vi "XNET.Settings.vi"(6 "Action":enum8{"Get", "Set"}(ring), 8 "error in (no error)":errorcluster, 10 "J1939 XNET Settings":T1={"Database"="", "Cluster"="", "Port"="", "Baud rate [Bd]"=500000, "Termination"=1, "Incoming Decimation"=1, "Outgoing Decimation"=1} {"Termination" items=["Off", "On"]}, 11 "Parent Ref in":T2 format="%.0x") -> (0 "error out":errorcluster, 2 "J1939 XNET Settings":T1={"Database"="", "Cluster"="", "Port"="", "Baud rate [Bd]"=0, "Termination"=0, "Incoming Decimation"=100, "Outgoing Decimation"=100} {"Termination" items=["Off", "On"]}, 3 "Item Ref out":T2 format="%.0x")   [LabVIEW 2019, in "J1939 Addon Shared.lvlib"]
uses:
  J1939 Addon Shared.lvlib
  Constants.vi
  <vilib>/NI VeriStand/Custom Device API/Custom Device API.lvlib
  <vilib>/NI VeriStand/Custom Device API/Get Item Property (String).vi
  <vilib>/NI VeriStand/Custom Device API/Get Item Property (U32).vi
  <vilib>/NI/NI VeriStand Advanced SysDef API/SysDef API/Advanced System Definition.lvlib
  <vilib>/NI/NI VeriStand Advanced SysDef API/_SubVIs/SysDef.Property.Set.String.vi
  <vilib>/NI/NI VeriStand Advanced SysDef API/_SubVIs/SysDef.Property.Set.U32.vi
  Types/XNET Settings.ctl
  <vilib>/NI VeriStand/Custom Device API/Custom Device Item Ref.ctl
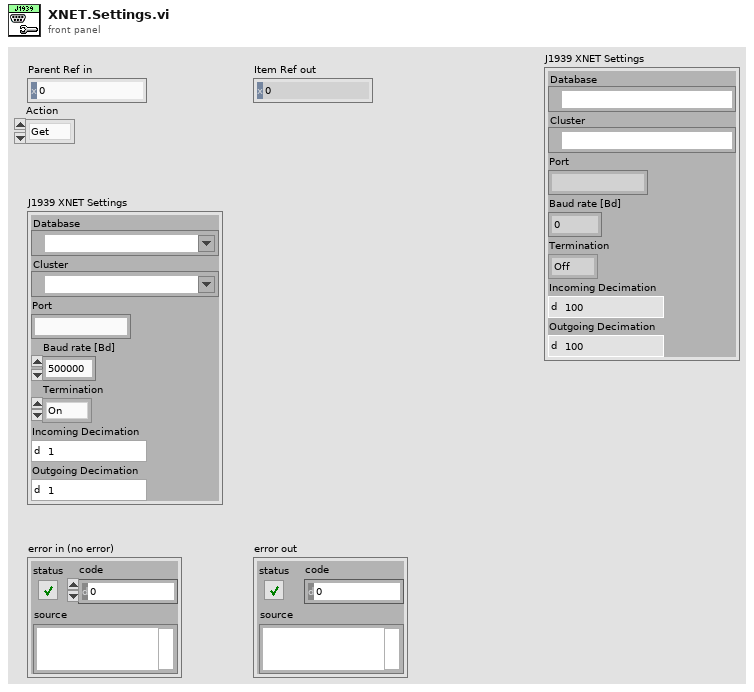
[diagram p1: front panel]
types:
  T1 = typedef "J1939 Addon Shared.lvlib/XNET Settings.ctl" = cluster{"Database":refnum<k21>, "Cluster":refnum<k21>, "Port":string, "Baud rate [Bd]":u32, "Termination":u32, "Incoming Decimation":u32, "Outgoing Decimation":u32}
  T2 = typedef "Custom Device API.lvlib/Custom Device Item Ref.ctl" = u64
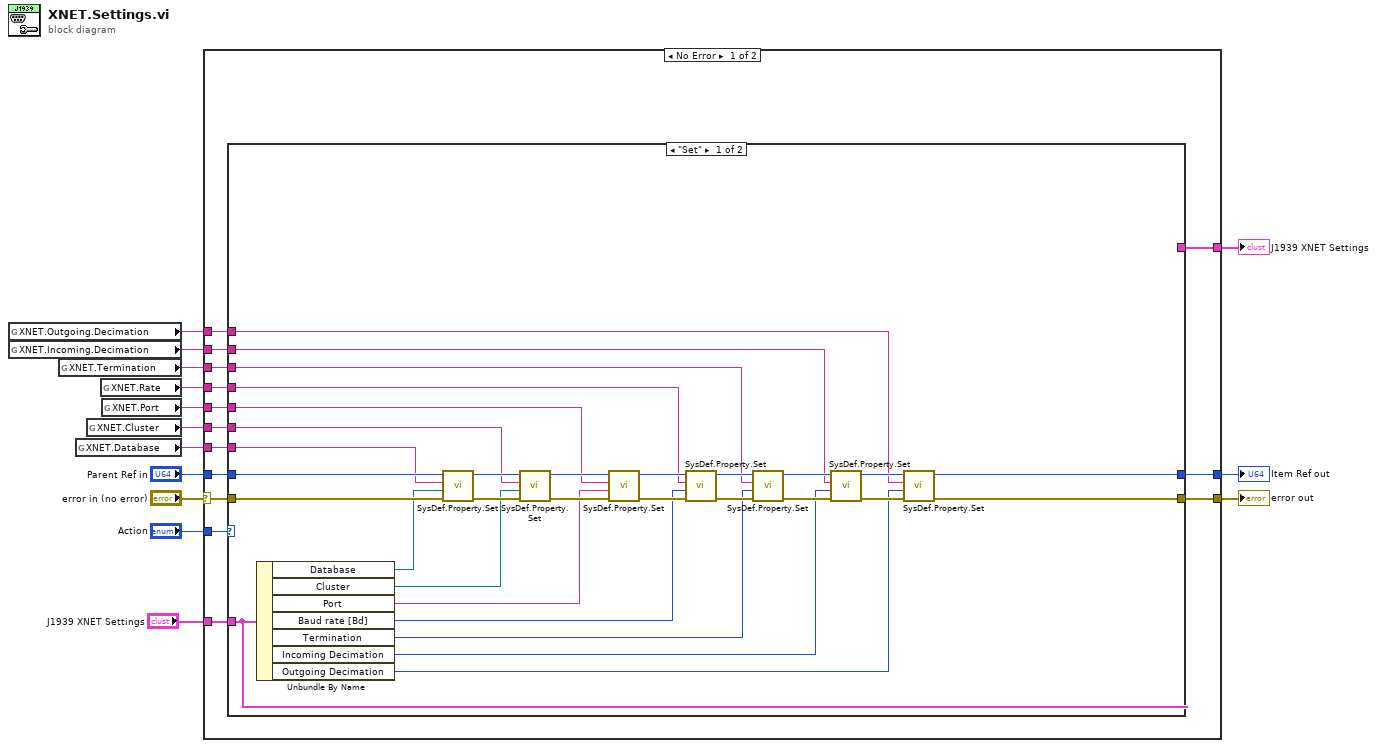
[diagram p0: block diagram]
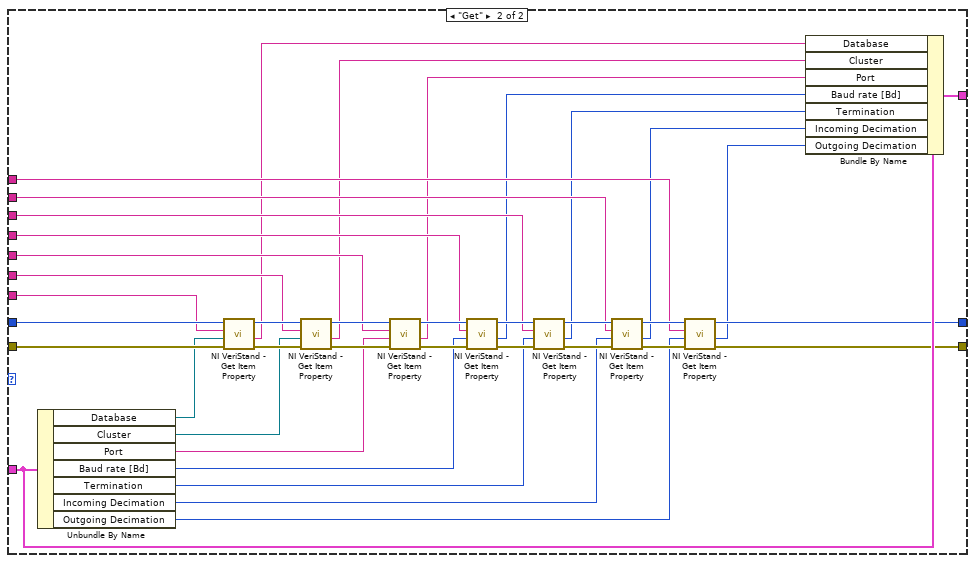
[diagram p2: hidden frame]
diagram:
  n1 = global read "Constants.vi" "XNET.Outgoing.Decimation"() -> (w7:string)
  n2 = global read "Constants.vi" "XNET.Incoming.Decimation"() -> (w6:string)
  n3 = global read "Constants.vi" "XNET.Termination"() -> (w5:string)
  n4 = global read "Constants.vi" "XNET.Database"() -> (w13:string)
  n5 = global read "Constants.vi" "XNET.Cluster"() -> (w9:string)
  n6 = global read "Constants.vi" "XNET.Rate"() -> (w4:string)
  n7 = global read "Constants.vi" "XNET.Port"() -> (w8:string)
  n8 = case shown="No Error" "error in (no error)" {
    selector: "error in (no error)" -> [w17 w101]
    tunnel: "Parent Ref in" -> [w28 w100]
    tunnel: w13 -> [w27 _]
    tunnel: "J1939 XNET Settings" -> [w26 w99]
    tunnel: [w25 w101] -> w11
    tunnel: [w24 w100] -> w10
    tunnel: w9 -> [w23 _]
    tunnel: w8 -> [w22 _]
    tunnel: w7 -> [w21 _]
    tunnel: w6 -> [w20 _]
    tunnel: w5 -> [w19 _]
    tunnel: w4 -> [w18 _]
    tunnel: "Action" -> [w16 _]
    tunnel: [w15 w99] -> w1
    frame No Error {
      n9 = case shown="\"Set\"" w16 {
        tunnel: w28 -> [w59 w98]
        tunnel: w27 -> [w58 w97]
        tunnel: w26 -> [w32 w70]
        tunnel: [w30 w63] -> w25
        tunnel: [w29 w62] -> w24
        tunnel: w23 -> [w39 w84]
        tunnel: w22 -> [w38 w83]
        tunnel: w21 -> [w37 w82]
        tunnel: w20 -> [w36 w81]
        tunnel: w19 -> [w35 w80]
        tunnel: w18 -> [w34 w79]
        tunnel: w17 -> [w33 w78]
        tunnel: [w32 w64] -> w15
        frame "Set" {
          n10 = Unbundle By Name(w32) -> ("Database"=w31:refnum<k21>, "Cluster"=w45:refnum<k21>, "Port"=w44:string, "Baud rate [Bd]"=w43:u32, "Termination"=w42:u32, "Incoming Decimation"=w41:u32, "Outgoing Decimation"=w40:u32)
          n11 = call-poly <vilib>:"SysDef.Property.Set.vi"("error in (no error)"=w33, "Value"=w31, "Property Name"=w58, "nodeID"=w59) -> ("error out"=w55:errorcluster, "nodeID out"=w54:u64)  [unwired: 6 in]
          n12 = call-poly <vilib>:"SysDef.Property.Set.vi"("error in (no error)"=w55, "Value"=w45, "Property Name"=w39, "nodeID"=w54) -> ("error out"=w56:errorcluster, "nodeID out"=w57:u64)  [unwired: 6 in]
          n13 = call-poly <vilib>:"SysDef.Property.Set.vi"("error in (no error)"=w56, "Value"=w44, "Property Name"=w38, "nodeID"=w57) -> ("error out"=w47:errorcluster, "nodeID out"=w46:u64)  [unwired: 6 in]
          n14 = call-poly <vilib>:"SysDef.Property.Set.vi"("error in (no error)"=w47, "Value"=w43, "Property Name"=w34, "nodeID"=w46) -> ("error out"=w50:errorcluster, "nodeID out"=w53:u64)  [unwired: 6 in]
          n15 = call-poly <vilib>:"SysDef.Property.Set.vi"("error in (no error)"=w50, "Value"=w42, "Property Name"=w35, "nodeID"=w53) -> ("error out"=w49:errorcluster, "nodeID out"=w52:u64)  [unwired: 6 in]
          n16 = call-poly <vilib>:"SysDef.Property.Set.vi"("error in (no error)"=w49, "Value"=w41, "Property Name"=w36, "nodeID"=w52) -> ("error out"=w48:errorcluster, "nodeID out"=w51:u64)  [unwired: 6 in]
          n17 = call-poly <vilib>:"SysDef.Property.Set.vi"("error in (no error)"=w48, "Value"=w40, "Property Name"=w37, "nodeID"=w51) -> ("error out"=w30:errorcluster, "nodeID out"=w29:u64)  [unwired: 6 in]
        }
        frame "Get" {
          n18 = Unbundle By Name(w70) -> ("Database"=w77:refnum<k21>, "Cluster"=w76:refnum<k21>, "Port"=w75:string, "Baud rate [Bd]"=w74:u32, "Termination"=w73:u32, "Incoming Decimation"=w72:u32, "Outgoing Decimation"=w71:u32)
          n19 = call-poly <vilib>:"NI VeriStand - Get Item Property.vi"("error in (no error)"=w78, "Default Value"=w77, "Property Name"=w97, "Item Ref in"=w98) -> ("error out"=w94:errorcluster, "Value"=w69:string, "Item Ref out"=w93:T2)  [unwired: 4 in, 1 out]
          n20 = call-poly <vilib>:"NI VeriStand - Get Item Property.vi"("error in (no error)"=w94, "Default Value"=w76, "Property Name"=w84, "Item Ref in"=w93) -> ("error out"=w95:errorcluster, "Value"=w68:string, "Item Ref out"=w96:T2)  [unwired: 4 in, 1 out]
          n21 = call-poly <vilib>:"NI VeriStand - Get Item Property.vi"("error in (no error)"=w95, "Default Value"=w75, "Property Name"=w83, "Item Ref in"=w96) -> ("error out"=w86:errorcluster, "Value"=w67:string, "Item Ref out"=w85:T2)  [unwired: 4 in, 1 out]
          n22 = call-poly <vilib>:"NI VeriStand - Get Item Property.vi"("error in (no error)"=w86, "Default Value"=w74, "Property Name"=w79, "Item Ref in"=w85) -> ("error out"=w89:errorcluster, "Value"=w66:u32, "Item Ref out"=w92:T2)  [unwired: 4 in, 1 out]
          n23 = call-poly <vilib>:"NI VeriStand - Get Item Property.vi"("error in (no error)"=w89, "Default Value"=w73, "Property Name"=w80, "Item Ref in"=w92) -> ("error out"=w88:errorcluster, "Value"=w65:u32, "Item Ref out"=w91:T2)  [unwired: 4 in, 1 out]
          n24 = call-poly <vilib>:"NI VeriStand - Get Item Property.vi"("error in (no error)"=w88, "Default Value"=w72, "Property Name"=w81, "Item Ref in"=w91) -> ("error out"=w87:errorcluster, "Value"=w61:u32, "Item Ref out"=w90:T2)  [unwired: 4 in, 1 out]
          n25 = call-poly <vilib>:"NI VeriStand - Get Item Property.vi"("error in (no error)"=w87, "Default Value"=w71, "Property Name"=w82, "Item Ref in"=w90) -> ("error out"=w63:errorcluster, "Value"=w60:u32, "Item Ref out"=w62:T2)  [unwired: 4 in, 1 out]
          n26 = Bundle By Name(cluster=w70, "Database"=w69, "Cluster"=w68, "Port"=w67, "Baud rate [Bd]"=w66, "Termination"=w65, "Incoming Decimation"=w61, "Outgoing Decimation"=w60) -> (w64:T1)
        }
      }
    }
    frame Error {
    }
  }
  "Item Ref out" <- w10
  "error out" <- w11
  "J1939 XNET Settings" <- w1
